vi "ILABs_GetVI.vi"(2 "errorIn":errorcluster, 3 "path":string, 4 "appReference":refnum<vi>) -> (0 "errorOut":string, 1 "vi reference":refnum<vi>)   [LabVIEW 2009]
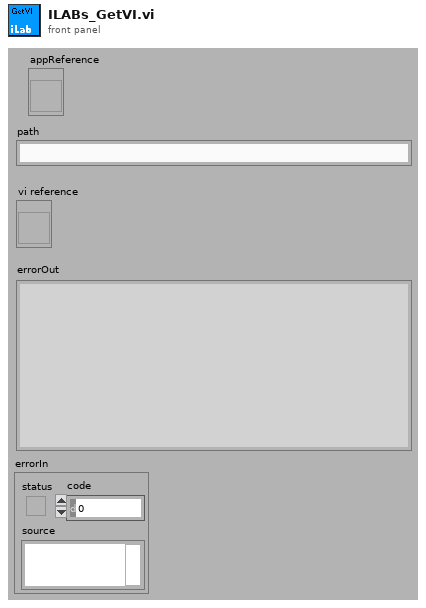
[diagram p1: front panel]
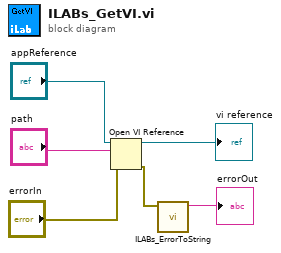
[diagram p0: block diagram]
diagram:
  n1 = Open VI Reference(application reference (local)="appReference", vi path="path", error in (no error)="errorIn") -> (vi reference=→"vi reference":refnum<vi>, error out=w5:errorcluster)  [unwired: 3 out]
  n2 = call "ILABs_ErrorToString.vi"("errorIn"=w5) -> ("errorOut"=→"errorOut":string)  [unwired: 10 out]
